vi "Main.vi"() -> ()   [LabVIEW 2021, in "Context.lvclass"]
uses:
  Context.lvclass
  A Context State/A Context State.lvclass
  C:/PPLs/Design-Patterns/State Pattern/State Pattern/State Pattern.lvclass
  B Context State/B Context State.lvclass
  Context.lvclass/Context.ctl
panel:
  out "Context I32 2":i32
  out "Context I32 1":i32
  # "Overview: Demonstrates the use of State Pattern using composition and AF messages. Context.lvlib is an Actor library that uses the state pattern. Composed State Pattern.lvlib is the library used to aid in developing the state pattern, with precreated State Transition.vi message along with logic to determine if a state may be transitioned into. All classes have unique colors and corresponding colored wires. This makes for easily seeing which common parent class exists on the block diagram.\n\nInstructions:\n1. View -> Bookmark Manager. Open the three #Demo bookmarks, keep their front panels open. Close their block diagrams.\n2. Before running this VI, note that the first state is transitioned into (Numeric) here using the State Transition.vi before Launch Root Actor. Subsequent state transitions occur by use of the front panel buttons. The states below implement that state transition. Closing the front panel Exits the current state.\n3. State messages are executed by use of the front panel buttons. The states below implement that message.\n2. Run this VI."
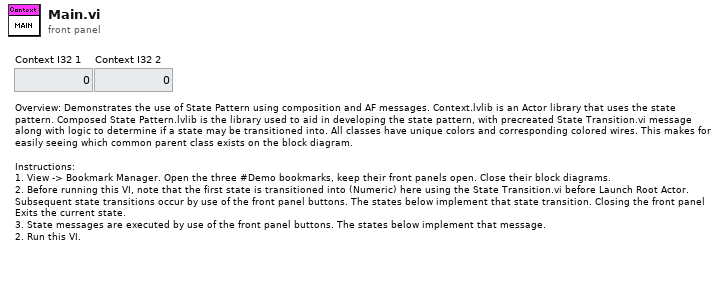
[diagram p1: front panel]
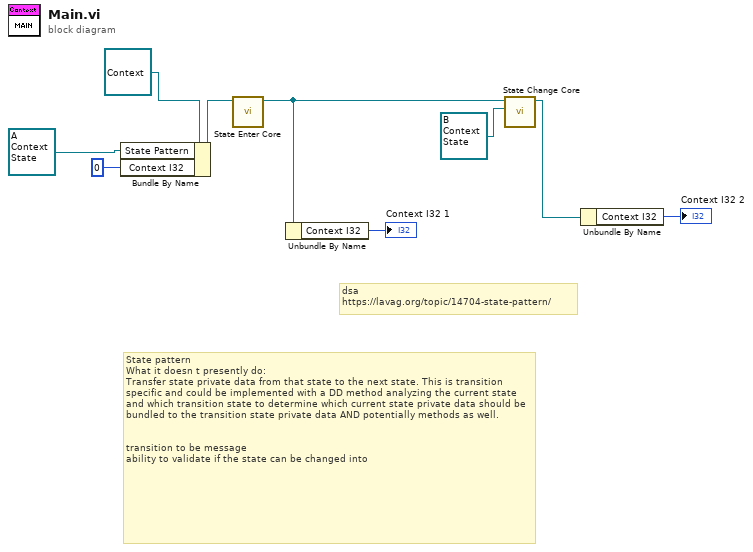
[diagram p0: block diagram]
diagram:
  # "State pattern\nWhat it doesn t presently do:\nTransfer state private data from that state to the next state. This is transition specific and could be implemented with a DD method analyzing the current state and which transition state to determine which current state private data should be bundled to the transition state private data AND potentially methods as well.\n\n\ntransition to be message\nability to validate if the state can be changed into"
  # "dsa\nhttps://lavag.org/topic/14704-state-pattern/"
  n1 = Bundle By Name(cluster=refnum<class "Context.lvclass"> refnum ("Context.lvclass"), "State Pattern"=refnum<class "A Context State.lvclass"> refnum ("A Context State.lvclass"), "Context I32"=0) -> (w4:refnum<class "Context.lvclass">)
  n2 = call-dynamic "State Enter Core.vi"("Context in"=w4) -> ("Context out"=w3:refnum<class "Context.lvclass">)  [unwired: 9 in, 1 out]
  n3 = Unbundle By Name(w3) -> ("Context I32"=→"Context I32 1":i32)
  n4 = call-dynamic "State Change Core.vi"("Transition State"=refnum<class "B Context State.lvclass"> refnum ("B Context State.lvclass"), "Context in"=w3) -> ("Context out"=w2:refnum<class "Context.lvclass">)  [unwired: 8 in, 1 out]
  n5 = Unbundle By Name(w2) -> ("Context I32"=→"Context I32 2":i32)
